vi "ReadLine.vi"(8 "Uart Input":cluster{u64}={185291944} {"?" format="%x"}, 10 "Buffer Size (32 bytes)":u32=64, 11 "Error Input":errorcluster) -> (0 "Uart Output":cluster{u64}={185291944} {"?" format="%x"}, 1 "Line String Buffer":string, 2 "Line String":string, 3 "Error Output":errorcluster, 4 "Line Bytes Buffer":u8[](array[numeric])=[69, 67, 67, 45, 76, 97, 98, 46, 0, 0, 0, 0, 0, 0, 0, 0, 0, 0, 0, 0, 0, 0, 0, 0, 0, 0, 0, 0, 0, 0, 0, 0, 0, 0, 0, 0, 0, 0, 0, 0, 0, 0, 0, 0, 0, 0, 0, 0, 0, 0, 0, 0, 0, 0, 0, 0, 0, 0, 0, 0, 0, 0, 0, 0] format="%x")   [LabVIEW 2019]
doc: "<B>Read</B> a received line from internal line buffer. The internal line buffer will be cleared. The <B>ReadLine</B> should be placed in the <B>Uart Line Event</B> case of an event structure."
uses:
  dll/LabViewUart.dll
panel:
  # "Read Line Buffer"
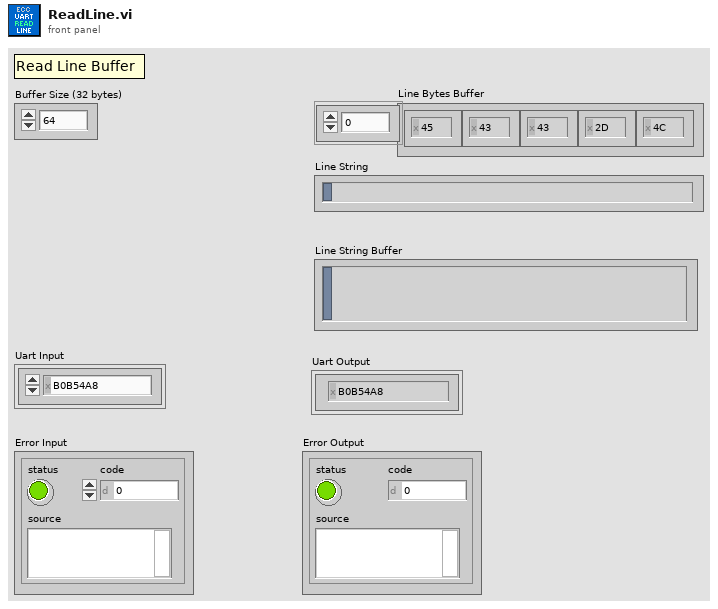
[diagram p1: front panel]
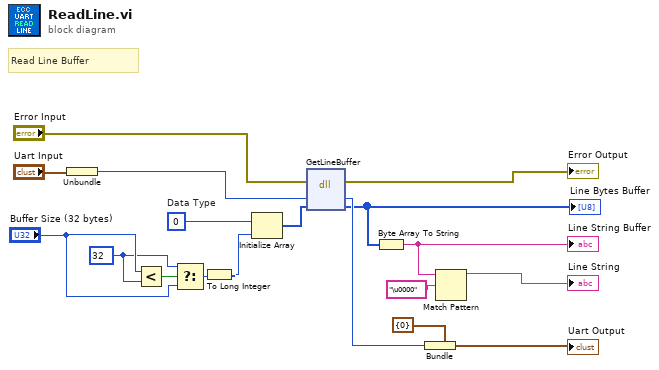
[diagram p0: block diagram]
diagram:
  w17 = u32 32 ("y")
  w11 = u8 0  # Data Type
  # "Read Line Buffer"
  n1 = Unbundle("Uart Input") -> (w8:u64)
  n2 = Less?(x="Buffer Size (32 bytes)", y=w17) -> (x < y?=w16:bool)
  n3 = Select(t=w17, s=w16, f="Buffer Size (32 bytes)") -> (s? t:f=w3:u32)
  n4 = To Long Integer(number=w3) -> (32bit integer=w2:i32)
  n5 = Initialize Array(w11, w2) -> (w12:u8[])
  n6 = dll-call lib="D:/Google Drive/INC-2020/INC352/INC352-2020/LabVIEW/examples/uart-cmdex/SubVI/dll/LabViewUart.dll" fn="GetLineBuffer"(error in="Error Input", "Object Handle"=w8, "Byte Buffer"=w12) -> (error out=→"Error Output":errorcluster, "Object Handle"=w6:u64, "Byte Buffer"=w1:u8[])  [unwired: 3 in, 1 out]
  "Line Bytes Buffer" <- w1
  n7 = Byte Array To String(unsigned byte array=w1) -> (string=w15:string)
  "Line String Buffer" <- w15
  n8 = Bundle(cluster=cluster{u64} {0}, w6) -> (→"Uart Output":cluster{u64})
  n9 = Match Pattern(string=w15, regular expression="\u0000") -> (before substring=→"Line String":string)  [unwired: 1 in, 3 out]
